vi "simple stepper.vi"(8 "error in (no error)":errorcluster, 10 "Forward? (TRUE)":bool) -> (0 "error out":errorcluster, 1 "Coil charge":bool[](array[boolean]), 3 "position":i32)   [LabVIEW 2009]
panel:
  # "ON is positive\nOFF is negative"
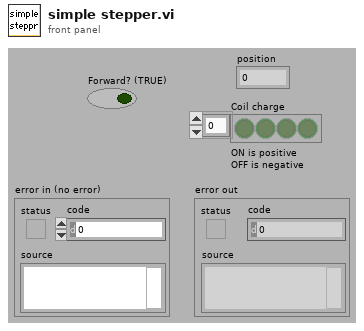
[diagram p1: front panel]
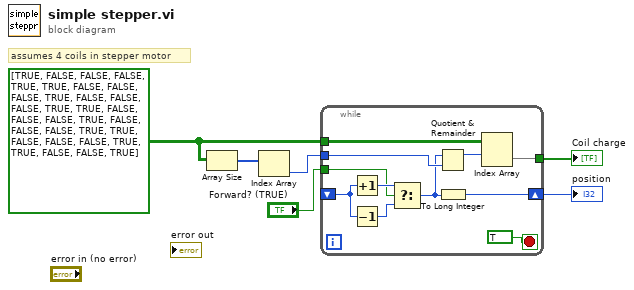
[diagram p0: block diagram]
diagram:
  w1 = bool[][] [[TRUE, FALSE, FALSE, FALSE], [TRUE, TRUE, FALSE, FALSE], [FALSE, TRUE, FALSE, FALSE], [FALSE, TRUE, TRUE, FALSE], [FALSE, FALSE, TRUE, FALSE], [FALSE, FALSE, TRUE, TRUE], [FALSE, FALSE, FALSE, TRUE], [TRUE, FALSE, FALSE, TRUE]] ("Coil charge")
  # "assumes 4 coils in stepper motor"
  n1 = Array Size(array=w1) -> (size(s)=w2:i32[])
  n2 = Index Array(array=w2) -> (element=w3:i32)  [unwired: 1 in]
  n3 = while {
    tunnel: w1 -> [w17]
    tunnel: w3 -> [w16]
    tunnel: [w14] -> w4
    shift-right: [w12] -> w5
    shift-left: _ -> [w11]
    tunnel: "Forward? (TRUE)" -> [w8]
    stop <- TRUE stop-if-true
    n4 = Increment(x=w11) -> (x+1=w10:i32)
    n5 = Decrement(x=w11) -> (x-1=w9:i32)
    n6 = Select(t=w10, s=w8, f=w9) -> (s? t:f=w7:i32)
    n7 = Quotient & Remainder(x=w7, y=w16) -> (x-y*floor(x/y)=w13:i32)  [unwired: 1 out]
    n8 = To Long Integer(number=w7) -> (32bit integer=w12:i32)
    n9 = Index Array(array=w17, index (row)=w13) -> (element=w14:bool[])  [unwired: 1 in]
  }
  "position" <- w5
  "Coil charge" <- w4
